vi "SRV_Read System Config File.vi"(0 "System Config File Path":path, 5 "start path  (Not A Path)":path=path "", 11 "error in (no error)":errorcluster) -> (4 "System Config File Path out":path, 8 "System Config":T1={"SRV IP Address"="", "Video Stream Rate Period (ms)"=250, "Enable Diagnostic Log"=FALSE, "Watchdog 1 Config"={"Watchdog Name"="", "Watchdog Period (s)"=1.0, "Watchdog Command"={"I2C Address"=0, "Register"=0, "Value"=0, "Active"=FALSE}}, "Watchdog 2 Config"={"Watchdog Name"="", "Watchdog Period (s)"=1.0, "Watchdog Command"={"I2C Address"=0, "Register"=0, "Value"=0, "Active"=FALSE}}, "Sensor Window Filepath"=path ""} {"Watchdog 2 Config"."Watchdog Period (s)" format="%.3f"; "Watchdog 2 Config"."Watchdog Command"."Value" format="%02x"; "Watchdog 2 Config"."Watchdog Command"."Register" format="%02x"; "Watchdog 2 Config"."Watchdog Command"."I2C Address" format="%02x"; "Watchdog 1 Config"."Watchdog Period (s)" format="%.3f"; "Watchdog 1 Config"."Watchdog Command"."Value" format="%02x"; "Watchdog 1 Config"."Watchdog Command"."Register" format="%02x"; "Watchdog 1 Config"."Watchdog Command"."I2C Address" format="%02x"}, 10 "Cancelled?":bool, 15 "error out":errorcluster)   [LabVIEW 2014]
uses:
  SRV_System Config.ctl
  Watchdog/SRV_Watchdog Config Cluster.ctl
  Motors/Motors Config/SRV_Motor Control Command Config.ctl
panel:
  # "I2C Address"
  # "Register"
  # "Value"
  # "Active"
  # "I2C Address"
  # "Register"
  # "Value"
  # "Active"
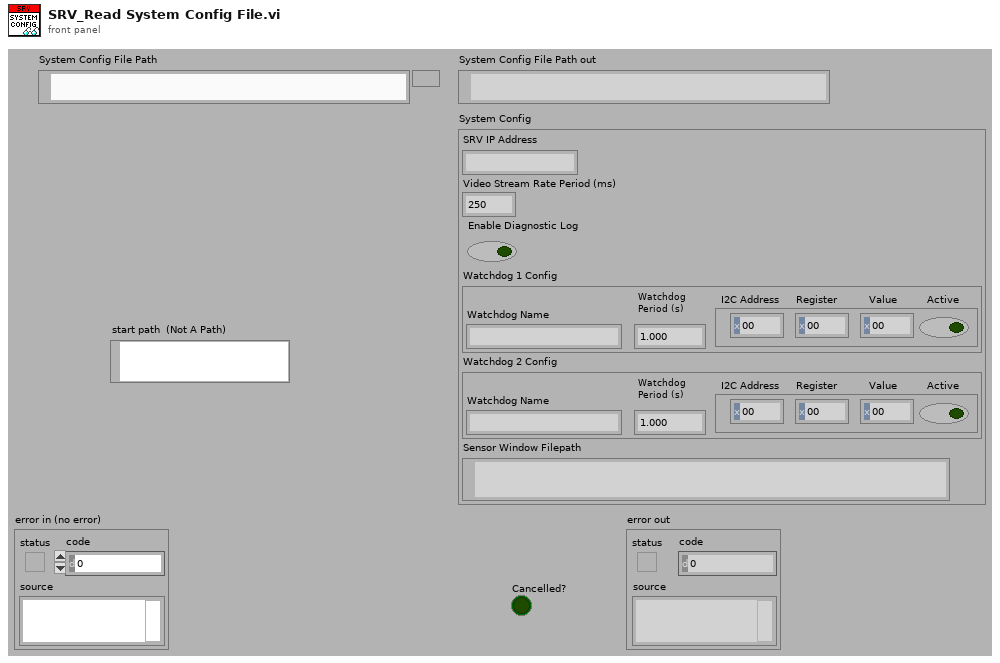
[diagram p1: front panel]
types:
  T1 = typedef "SRV_System Config.ctl" = cluster{"SRV IP Address":string, "Video Stream Rate Period (ms)":u32, "Enable Diagnostic Log":bool, "Watchdog 1 Config":T2, "Watchdog 2 Config":T2, "Sensor Window Filepath":path}
  T2 = typedef "SRV_Watchdog Config Cluster.ctl" = cluster{"Watchdog Name":string, "Watchdog Period (s)":dbl, "Watchdog Command":T3}
  T3 = typedef "SRV_Motor Control Command Config.ctl" = cluster{"I2C Address":u8, "Register":u8, "Value":u8, "Active":bool}
  T4 = enum16{"open", "open or create", "create or replace", "create", "open (read only)"}
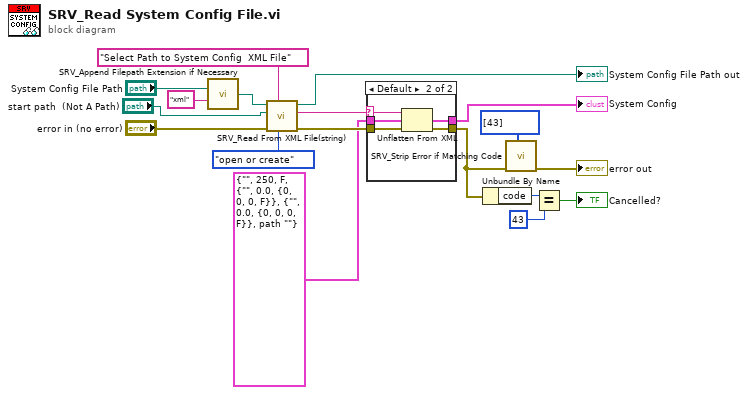
[diagram p0: block diagram]
diagram:
  n1 = call "SRV_Append Filepath Extension if Necessary.vi"("Filepath"="System Config File Path", "Extension"="xml") -> ("Filepath with Extension"=w10:path)  [unwired: 13 in]
  n2 = call "SRV_Read From XML File(string).vi"("function (open-read-only:4)"=T4."open or create", "Prompt"="Select Path to System Config  XML File", "error in (no error)"="error in (no error)", "start path  (Not A Path)"="start path  (Not A Path)", "XML File Path"=w10) -> ("error out"=w12:errorcluster, "XML Elements"=w8:string, "XML File Path(duplicate)"=→"System Config File Path out":path)  [unwired: 4 in]
  n3 = case shown="Default" w8 {
    selector: w8 -> [_ w21]
    tunnel: T1 {"SRV IP Address"="", "Video Stream Rate Period (ms)"=250, "Enable Diagnostic Log"=FALSE, "Watchdog 1 Config"={"Watchdog Name"="", "Watchdog Period (s)"=0.0, "Watchdog Command"={"I2C Address"=0, "Register"=0, "Value"=0, "Active"=FALSE}}, "Watchdog 2 Config"={"Watchdog Name"="", "Watchdog Period (s)"=0.0, "Watchdog Command"={"I2C Address"=0, "Register"=0, "Value"=0, "Active"=FALSE}}, "Sensor Window Filepath"=path ""} ("System Config") -> [w19 w25]
    tunnel: [w19 w24] -> w6
    tunnel: [w20 w23] -> w4
    tunnel: w12 -> [w20 w22]
    frame "" {
    }
    frame Default {
      n4 = Unflatten From XML(xml string=w21, type=w25, error in (no error)=w22) -> (value=w24:T1, error out=w23:errorcluster)
    }
  }
  "System Config" <- w6
  n5 = Unbundle By Name(w4) -> ("code"=w16:i32)
  n6 = call "SRV_Strip Error if Matching Code.vi"("error in (no error)"=w4, "Strip Codes"=i32[] [43]) -> ("error out"=→"error out":errorcluster)  [unwired: 8 in]
  n7 = Equal?(x=w16, y=43) -> (x = y?=→"Cancelled?":bool)
